vi "VDH-RequestSaveData.vi"(8 "error in (no error)":errorcluster, 10 "Save Parameters":T1={"Size in sets (0=Until stop)"=1, "Folder Path"=path "", "filename"=""}, 11 "VDH-VNA_data_handler in":refnum<class "VDH-VNA_data_handler.lvclass">) -> (0 "error out":errorcluster, 3 "VDH-VNA_data_handler out":refnum<class "VDH-VNA_data_handler.lvclass">)   [LabVIEW 2020, in "VDH-VNA_data_handler.lvlib" / "VDH-VNA_data_handler.lvclass"]
uses:
  VDH-VNA_data_handler.lvclass
  VDH-save_parameters.ctl
  VDH-VNA_data_handler.lvclass/VDH-VNA_data_handler.ctl
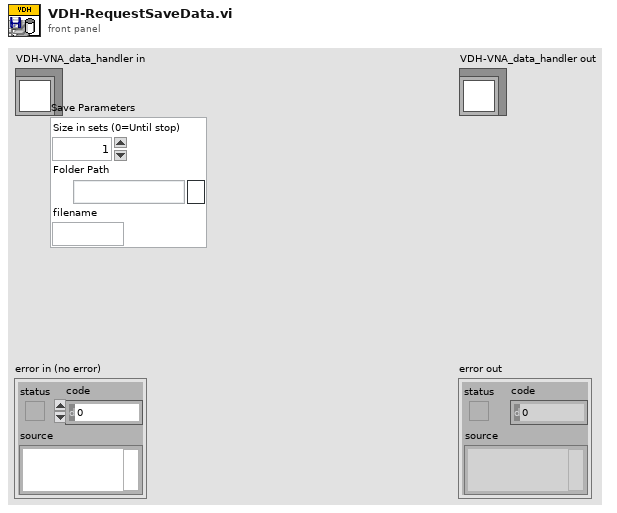
[diagram p1: front panel]
types:
  T1 = typedef "VDH-VNA_data_handler.lvlib/VDH-VNA_data_handler.lvclass/VDH-save_parameters.ctl" = cluster{"Size in sets (0=Until stop)":u8, "Folder Path":path, "filename":string}
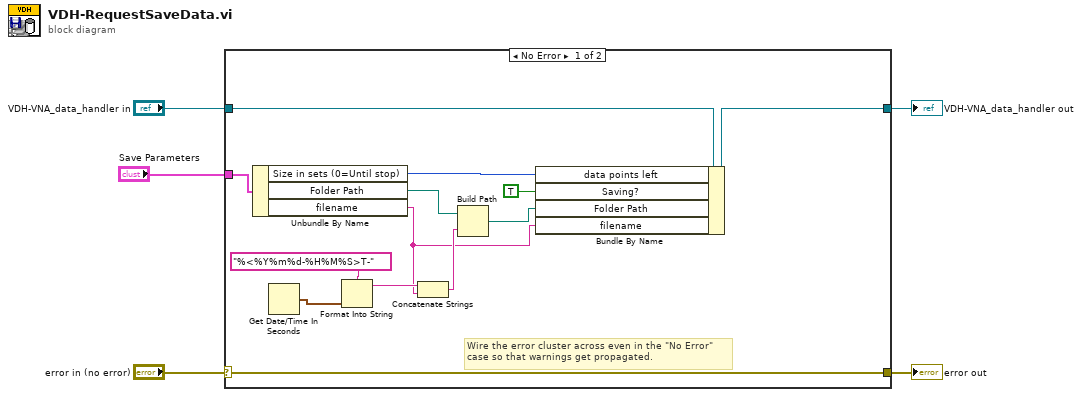
[diagram p0: block diagram]
diagram:
  n1 = case shown="No Error" "error in (no error)" {
    selector: "error in (no error)" -> [w18 w20]
    tunnel: [w18 w20] -> w4
    tunnel: [w16 w19] -> w2
    tunnel: "VDH-VNA_data_handler in" -> [w17 w19]
    tunnel: "Save Parameters" -> [w15 _]
    frame No Error {
      # "Wire the error cluster across even in the \"No Error\"\ncase so that warnings get propagated."
      n2 = Unbundle By Name(w15) -> ("Size in sets (0=Until stop)"=w14:u8, "Folder Path"=w12:path, "filename"=w6:string)
      n3 = Get Date/Time In Seconds() -> (seconds since 1Jan1904=w10:timestamp)
      n4 = Format Into String(format string="%<%Y%m%d-%H%M%S>T-", w10) -> (resulting string=w9:string)  [unwired: 2 in, 1 out]
      n5 = Concatenate Strings(w9, w6) -> (w8:string)
      n6 = Build Path(base path=w12, name or relative path=w8) -> (appended path=w7:path)
      n7 = Bundle By Name(cluster=w17, "data points left"=w14, "Saving?"=TRUE ("data saving info.Saving?"), "Folder Path"=w7, "filename"=w6) -> (w16:refnum<class "VDH-VNA_data_handler.lvclass">)
    }
    frame Error {
    }
  }
  "error out" <- w4
  "VDH-VNA_data_handler out" <- w2
